vi "LSCI 370 Config Resistance Range.vi"(0 "VISA session":refnum<visa-resource-name>, 1 "Autorange (F: Autorange OFF)":bool, 2 "Excitation On/Off (T: Excitation ON)":bool=TRUE, 5 "Channel (1)":i32=1 min=0 max=16 step=1, 7 "Excitation Mode (0: Voltage)":u16(ring) items=["Voltage", "Current"], 9 "Excitation Range (11: 632 mV / 316 nA)":u16(ring)=11 items=["2.00 uV / 1.00 pA", "6.32 uV / 3.16 pA", "20.0 uV / 10.0 pA", "63.2 uV / 31.6 pA", "200 uV / 100 pA", "632 uV / 316 pA", "2.00 mV / 1.00 nA", "6.32 mV / 3.16 nA", "20.0 mV / 10.0 nA", "63.2 mV / 31.6 nA", "200 mV / 100 nA", "632 mV / 316 nA", "1.00 uA", "3.16 uA", "10.0 uA", "31.6 uA", "100 uA", "316 uA", "1.00 mA", "3.16 mA", "10.0 mA", "31.6 mA"], 11 "error in (no error)":errorcluster, 12 "Resistance Range (21: 63.2 MOhm)":u16(ring)=21 items=["2.00 mOhm", "6.32 mOhm", "20.0 mOhm", "63.2 mOhm", "200 mOhm", "632 mOhm", "2.00 Ohm", "6.32 Ohm", "20.0 Ohm", "63.2 Ohm", "200 Ohm", "632 Ohm", "2.00 kOhm", "6.32 kOhm", "20.0 kOhm", "63.2 kOhm", "200 kOhm", "632 kOhm", "2.00 MOhm", "6.32 MOhm", "20.0 MOhm", "63.2 MOhm"]) -> (4 "dup VISA session":refnum<visa-resource-name>, 15 "error out":errorcluster)   [LabVIEW 2016]
doc: "This VI configures the Excitation Modes, Resistance Range, and Autorange."
panel:
  # "Autorange ON\nAutorange OFF"
  # "Excitation ON\nExcitation OFF"
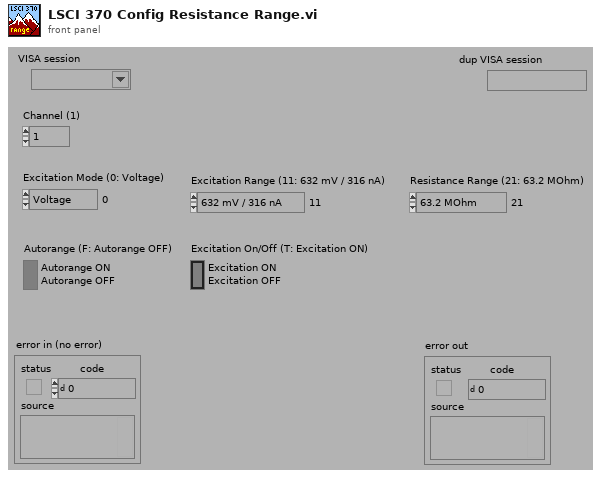
[diagram p1: front panel]
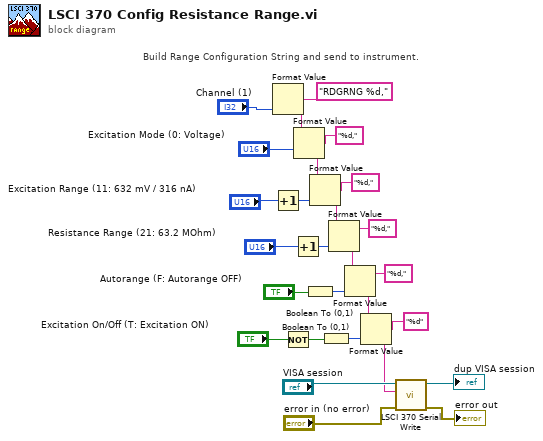
[diagram p0: block diagram]
diagram:
  # "Build Range Configuration String and send to instrument."
  n1 = Format Value(format string="RDGRNG %d,", value (0)="Channel (1)") -> (output string=w16:string)  [unwired: 1 in]
  n2 = Increment(x="Excitation Range (11: 632 mV / 316 nA)") -> (x+1=w9:u16)
  n3 = Not(x="Excitation On/Off (T: Excitation ON)") -> (.not. x?=w1:bool)
  n4 = Increment(x="Resistance Range (21: 63.2 MOhm)") -> (x+1=w8:u16)
  n5 = Format Value(string ("")=w16, format string="%d,", value (0)="Excitation Mode (0: Voltage)") -> (output string=w15:string)
  n6 = Boolean To (0,1)(Boolean="Autorange (F: Autorange OFF)") -> (0, 1=w3:i16)
  n7 = Format Value(string ("")=w15, format string="%d,", value (0)=w9) -> (output string=w20:string)
  n8 = Boolean To (0,1)(Boolean=w1) -> (0, 1=w2:i16)
  n9 = Format Value(string ("")=w20, format string="%d,", value (0)=w8) -> (output string=w13:string)
  n10 = Format Value(string ("")=w13, format string="%d,", value (0)=w3) -> (output string=w12:string)
  n11 = Format Value(string ("")=w12, format string="%d", value (0)=w2) -> (output string=w19:string)
  n12 = call "LSCI 370 Serial Write.vi"("error in (no error)"="error in (no error)", "Write Buffer (\"\")"=w19, "VISA session"="VISA session") -> ("error out"=→"error out":errorcluster, "dup VISA session"=→"dup VISA session":refnum<visa-resource-name>)  [unwired: 6 in, 1 out]
